vi "T02 - опрос характеристик устройства.vi"() -> ()   [LabVIEW 2009]
uses:
  Z210/Z210 CTL Lib.llb/Z210 CTL ADC or DAC Function.ctl
panel:
  in  "stop":bool
  out "Common Parameters":T1
  in  "AorD":T2
  # "Можно узнать основные параметры АЦП/ЦАП: число выводов,\nразрешение, вес наименьшего разряда и размер отсчета."
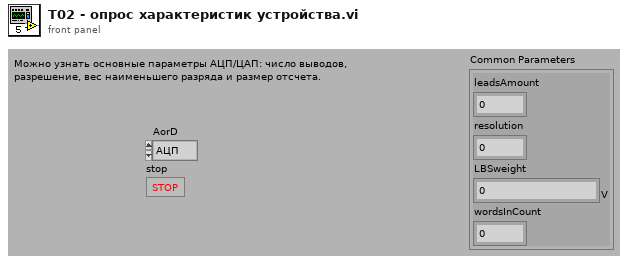
[diagram p1: front panel]
types:
  T1 = cluster{"leadsAmount":i32, "resolution":i32, "LBSweight":dbl[unit], "wordsInCount":i32}
  T2 = typedef "Z210 CTL ADC or DAC Function.ctl" = enum16{"АЦП", "ЦАП", "Both"}
  T3 = typedef "Z210 CTL Unit Data .ctl" = cluster{"typeDevice":i32, "numberDSP":i32}
  T4 = cluster{"inputsAmount":i32, "resolution":i32, "LBSweight":dbl[unit], "wordsInCount":i32}
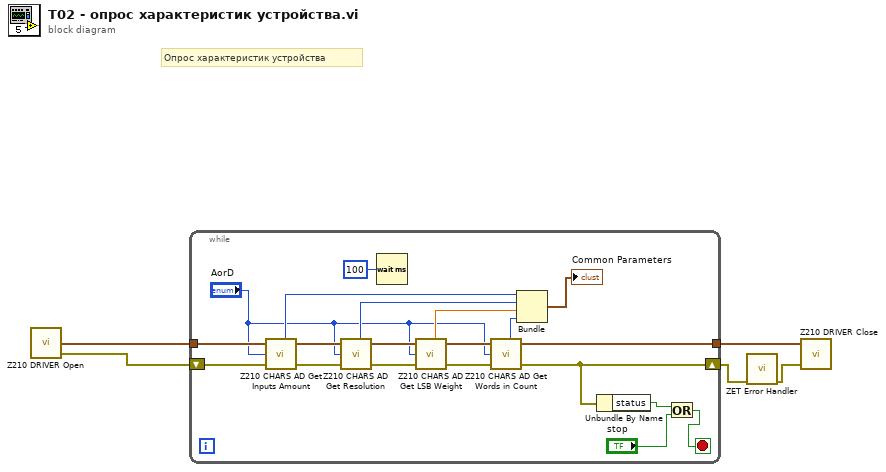
[diagram p0: block diagram]
diagram:
  # "Опрос характеристик устройства"
  n1 = call "Z210 DRIVER Open.vi"() -> ("unitData out"=w3:T3, "error IO"=w4:errorcluster)  [unwired: 8 in]
  n2 = while {
    tunnel: w3 -> [w12]
    tunnel: [w9] -> w2
    shift-right: [w8] -> w1
    shift-left: w4 -> [w13]
    stop <- w24 stop-if-true
    n3 = call "Z210 CHARS AD Get Inputs Amount.vi"("unitData in"=w12, "AorD"="AorD", "error in (no error)"=w13) -> ("inputsAmount"=w20:i32, "unitData out"=w14:T3, "error out"=w17:errorcluster)  [unwired: 4 in]
    n4 = call "Z210 CHARS AD Get Resolution.vi"("unitData in"=w14, "AorD"="AorD", "error in (no error)"=w17) -> ("resolution"=w21:i32, "unitData out"=w15:T3, "error out"=w18:errorcluster)  [unwired: 4 in]
    n5 = Wait (ms)(milliseconds to wait=u32 100) -> ()  [unwired: 1 out]
    n6 = call "Z210 CHARS AD Get LSB Weight.vi"("unitData in"=w15, "AorD"="AorD", "error in (no error)"=w18) -> ("LBSweight"=w22:dbl[unit], "unitData out"=w16:T3, "error out"=w19:errorcluster)  [unwired: 4 in]
    n7 = call "Z210 CHARS AD Get Words in Count.vi"("unitData in"=w16, "AorD"="AorD", "error in \n(no error)"=w19) -> ("wordsInCount"=w23:i32, "unitData out"=w9:T3, "error out"=w8:errorcluster)  [unwired: 4 in]
    n8 = Bundle("inputsAmount"=w20, "resolution"=w21, "LBSweight"=w22, "wordsInCount"=w23) -> (→"Common Parameters":T4)  [unwired: 1 in]
    n9 = Unbundle By Name(w8) -> ("status"=w7:bool)
    n10 = Or(x=w7, y="stop") -> (x .or. y?=w24:bool)
  }
  n11 = call "ZET Error Handler.vi"("error in (no error)"=w1) -> ("error out"=w5:errorcluster)  [unwired: 9 in, 1 out]
  n12 = call "Z210 DRIVER Close.vi"("unitData in"=w2, "error in (no error)"=w5) -> ()  [unwired: 6 in, 2 out]
